vi "多脉冲测试脚本.vi"(1 "测试参数":cluster{"参数值":dbl[], "时序优先":bool, "4-wire":bool}) -> (0 "Script":string)   [LabVIEW 2020]
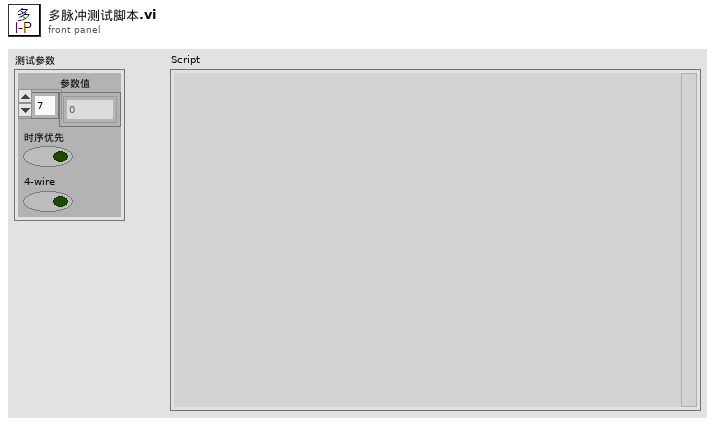
[diagram p1: front panel]
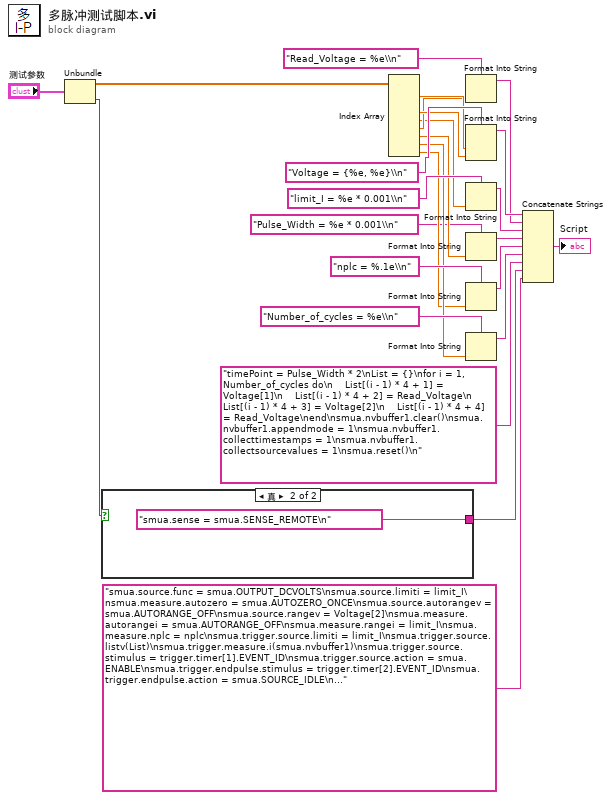
[diagram p0: block diagram]
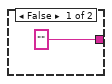
[diagram p2: hidden frame]
diagram:
  n1 = Unbundle("测试参数") -> ("参数值"=w9:dbl[], "4-wire"=w10:bool)  [unwired: 1 out]
  n2 = case shown="真" w10 {
    tunnel: ["" "smua.sense = smua.SENSE_REMOTE\n"] -> w15
    frame False {
    }
    frame True {
    }
  }
  n3 = Index Array(array=w9) -> (element #1=w8:dbl, element #3=w7:dbl, element #4=w4:dbl, element #5=w6:dbl, element #6=w3:dbl, element #7=w5:dbl, element #8=w2:dbl)  [unwired: 8 in, 1 out]
  n4 = Format Into String(format string="Read_Voltage = %e\\n" ("格式字符串"), w6) -> (resulting string=w21:string)  [unwired: 2 in, 1 out]
  n5 = Format Into String(format string="Voltage = {%e, %e}\\n" ("格式字符串"), w8, w7) -> (resulting string=w23:string)  [unwired: 2 in, 1 out]
  n6 = Format Into String(format string="limit_I = %e * 0.001\\n" ("格式字符串"), w4) -> (resulting string=w20:string)  [unwired: 2 in, 1 out]
  n7 = Format Into String(format string="Pulse_Width = %e * 0.001\\n", w3) -> (resulting string=w19:string)  [unwired: 2 in, 1 out]
  n8 = Format Into String(format string="nplc = %.1e\\n", w2) -> (resulting string=w17:string)  [unwired: 2 in, 1 out]
  n9 = Format Into String(format string="Number_of_cycles = %e\\n" ("格式字符串"), w5) -> (resulting string=w12:string)  [unwired: 2 in, 1 out]
  n10 = Concatenate Strings(w23, w21, w20, w19, w17, w12, "timePoint = Pulse_Width * 2\nList = {}\nfor i = 1, Number_of_cycles do\n    List[(i - 1) * 4 + 1] = Voltage[1]\n    List[(i - 1) * 4 + 2] = Read_Voltage\n    List[(i - 1) * 4 + 3] = Voltage[2]\n    List[(i - 1) * 4 + 4] = Read_Voltage\nend\nsmua.nvbuffer1.clear()\nsmua.nvbuffer1.appendmode = 1\nsmua.nvbuffer1.collecttimestamps = 1\nsmua.nvbuffer1.collectsourcevalues = 1\nsmua.reset()\n", w15, "smua.source.func = smua.OUTPUT_DCVOLTS\nsmua.source.limiti = limit_I\nsmua.measure.autozero = smua.AUTOZERO_ONCE\nsmua.source.autorangev = smua.AUTORANGE_OFF\nsmua.source.rangev = Voltage[2]\nsmua.measure.autorangei = smua.AUTORANGE_OFF\nsmua.measure.rangei = limit_I\nsmua.measure.nplc = nplc\nsmua.trigger.source.limiti = limit_I\nsmua.trigger.source.listv(List)\nsmua.trigger.measure.i(smua.nvbuffer1)\nsmua.trigger.source.stimulus = trigger.timer[1].EVENT_ID\nsmua.trigger.source.action = smua.ENABLE\nsmua.trigger.endpulse.stimulus = trigger.timer[2].EVENT_ID\nsmua.trigger.endpulse.action = smua.SOURCE_IDLE\nsmua.trigger.measure.action = smua.ENABLE\nsmua.trigger.count = table.getn(List)\nsmua.trigger.arm.stimulus = trigger.EVENT_ID\ntrigger.timer[1].reset()\ntrigger.timer[1].stimulus = smua.trigger.ARMED_EVENT_ID\ntrigger.timer[1].passthrough = false\ntrigger.timer[1].delay = timePoint\ntrigger.timer[1].count = table.getn(List)\ntrigger.timer[2].reset()\ntrigger.timer[2].stimulus = trigger.timer[1].EVENT_ID\ntrigger.timer[2].passthrough = false\ntrigger.timer[2].delay = Pulse_Width\ntrigger.timer[2].count = 1\nsmua.source.output = smua.OUTPUT_ON\nsmua.trigger.initiate()\ndelay(1e-3)\nsmua.trigger.arm.set()\nwaitcomplete()\nsmua.source.leveli = 0\nsmua.source.levelv = 0\nsmua.source.output = smua.OUTPUT_OFF\nStart = 1\nStop = table.getn(List)\nprint(\"{\" .. Stop - Start + 1 .. \"}\")\nprintbuffer(Start, Stop, smua.nvbuffer1.timestamps)\nprintbuffer(Start, Stop, smua.nvbuffer1.sourcevalues)\nprintbuffer(Start, Stop, smua.nvbuffer1)\nprintbuffer(Start, Stop, smua.nvbuffer1.sourcevalues)\nprint(\"{done}\")\nreset()\n") -> (→"Script":string)
